vi "Set Arm.vi"(8 "error in (no error)":errorcluster, 9 "arm index":i32, 10 "youBot arm in":refnum<class "NI_Robotics_KUKA youBot Arm.lvclass">, 11 "youBot host in":refnum<class "NI_Robotics_KUKA youBot Host Interface.lvclass">) -> (0 "error out":errorcluster, 3 "youBot host out":refnum<class "NI_Robotics_KUKA youBot Host Interface.lvclass">)   [LabVIEW 2017, in "NI_Robotics_KUKA youBot Host.lvlib" / "NI_Robotics_KUKA youBot Host Interface.lvclass"]
uses:
  <vilib>/robotics/KUKA youBot/Host Interface/NI_Robotics_KUKA youBot Host Interface.lvclass
  <vilib>/robotics/KUKA youBot/Basic Device/Arm/NI_Robotics_KUKA youBot Arm.lvclass
  <vilib>/robotics/KUKA youBot/Host Interface/NI_Robotics_KUKA youBot Host Interface.lvclass/NI_Robotics_KUKA youBot Host Interface.ctl
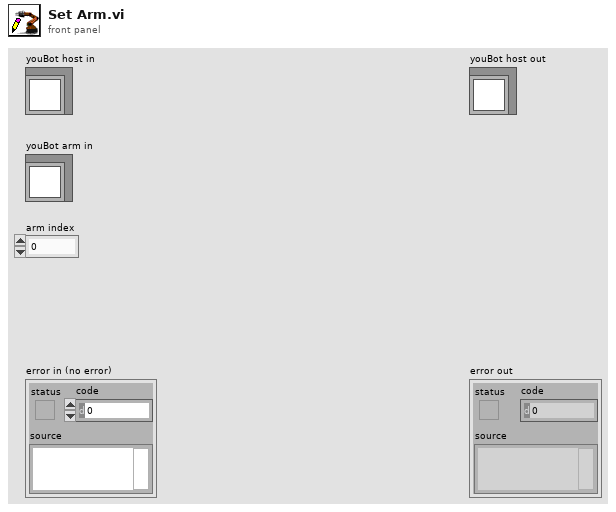
[diagram p1: front panel]
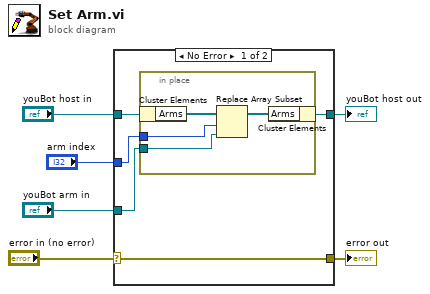
[diagram p0: block diagram]
diagram:
  n1 = case shown="No Error" "error in (no error)" {
    selector: "error in (no error)" -> [w11 w16]
    tunnel: [w11 w16] -> w5
    tunnel: [w7 w17] -> w3
    tunnel: "youBot host in" -> [w10 w17]
    tunnel: "youBot arm in" -> [w8 _]
    tunnel: "arm index" -> [w9 _]
    frame No Error {
      n2 = in-place {
        in-place-border: w9 -> [w14]
        in-place-border: w8 -> [w13]
        n3 = in-place-cluster #1(w10) -> ("Arms"=w15:refnum<class "NI_Robotics_KUKA youBot Arm.lvclass">[])
        n4 = Replace Array Subset(array=w15, new element=w13, index=w14) -> (w12:refnum<class "NI_Robotics_KUKA youBot Arm.lvclass">[])
        n5 = in-place-cluster #1("Arms"=w12) -> (w7:refnum<class "NI_Robotics_KUKA youBot Host Interface.lvclass">)
      }
    }
    frame Error {
    }
  }
  "error out" <- w5
  "youBot host out" <- w3
